vi "Trust Actual Server Identity.vi"(8 "error in (no error)":errorcluster, 10 "fingerprint":string, 11 "SSH Client in":refnum<class "OpenSSH Client.lvclass">) -> (0 "error out":errorcluster, 2 "permanent?":bool, 3 "SSH Client out":refnum<class "OpenSSH Client.lvclass">)   [LabVIEW 2020, in "NI_SSH.lvlib" / "OpenSSH Client.lvclass"]
uses:
  <vilib>/net/SSH/Client/OpenSSH/OpenSSH Client.lvclass
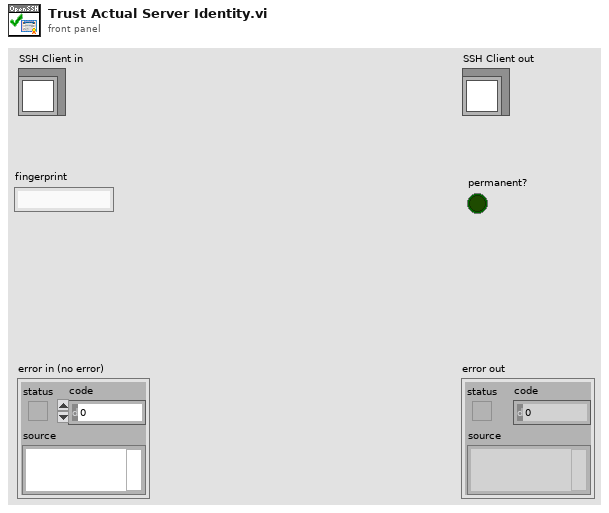
[diagram p1: front panel]
types:
  T1 = enum16{"open", "replace", "create", "open or create", "replace or create", "replace or create with confirmation"}
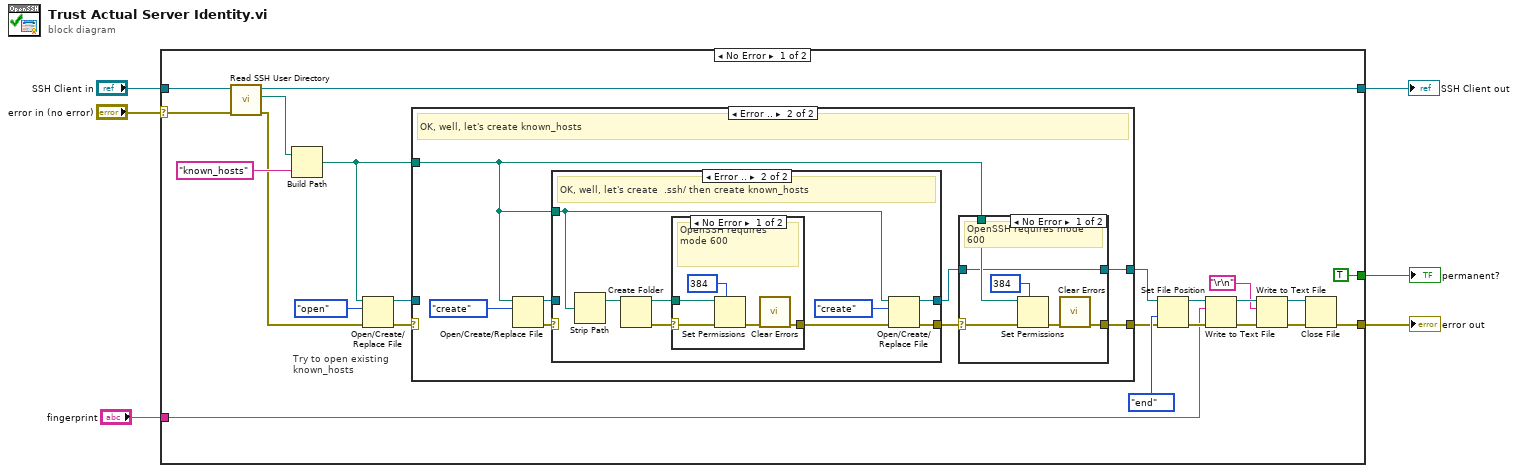
[diagram p0: block diagram]
diagram:
  n1 = case shown="No Error" "error in (no error)" {
    selector: "error in (no error)" -> [w28 w64]
    tunnel: "SSH Client in" -> [w29 w65]
    tunnel: "fingerprint" -> [w21 _]
    tunnel: [w15 w64] -> w3
    tunnel: [TRUE ("permanent?") _] -> w2
    tunnel: [w13 w65] -> w1
    frame No Error {
      # "Try to open existing known_hosts"
      n2 = call <vilib>:"Read SSH User Directory.vi"("error in (no error)"=w28, "OpenSSH Client in"=w29) -> ("error out"=w7:errorcluster, "Path"=w27:path, "OpenSSH Client out"=w13:refnum<class "OpenSSH Client.lvclass">)  [unwired: 7 in]
      n3 = Build Path(base path=w27, name or relative path="known_hosts") -> (appended path=w8:path)
      n4 = Open/Create/Replace File(file path (use dialog)=w8, error in=w7, operation (0:open)=T1."open") -> (refnum out=w11:refnum<file>, error out=w12:errorcluster)  [unwired: 3 in, 1 out]
      n5 = case shown="Error .." w12 {
        selector: w12 -> [w30 _]
        tunnel: w11 -> [w31 _]
        tunnel: [w31 w33] -> w9
        tunnel: [w30 w34] -> w10
        tunnel: w8 -> [_ w32]
        frame No Error {
        }
        frame Error {
          # "OK, well, let's create known_hosts"
          n6 = Open/Create/Replace File(file path (use dialog)=w32, operation (0:open)=T1."create") -> (refnum out=w37:refnum<file>, error out=w38:errorcluster)  [unwired: 4 in, 1 out]
          n7 = case shown="Error .." w38 {
            selector: w38 -> [w49 _]
            tunnel: [w49 w50] -> w35
            tunnel: w37 -> [w48 _]
            tunnel: [w48 w51] -> w36
            tunnel: w32 -> [_ w53]
            frame No Error {
            }
            frame Error {
              # "OK, well, let's create  .ssh/ then create known_hosts"
              n8 = Strip Path(path=w53) -> (stripped path=w57:path)  [unwired: 1 out]
              n9 = Create Folder(path (use dialog)=w57) -> (created path=w55:path, error out=w56:errorcluster)  [unwired: 2 in, 1 out]
              n10 = case shown="No Error" w56 {
                selector: w56 -> [w60 w63]
                tunnel: w55 -> [w61 _]
                tunnel: [w58 w63] -> w54
                frame No Error {
                  # "OpenSSH requires mode 600"
                  n11 = Set Permissions(7:i16 384 ("permissions"), 8:w60, 11:w61) -> (0:w59:errorcluster)  [unwired: 2 in, 1 out]
                  n12 = call <vilib>:"Clear Errors.vi"("error in (no error)"=w59) -> ("error out"=w58:errorcluster)  [unwired: 5 in, 1 out]
                }
                frame Error {
                  # "Well, phooey"
                }
              }
              n13 = Open/Create/Replace File(file path (use dialog)=w53, error in=w54, operation (0:open)=T1."create") -> (refnum out=w51:refnum<file>, error out=w50:errorcluster)  [unwired: 3 in, 1 out]
            }
          }
          n14 = case shown="No Error" w35 {
            selector: w35 -> [w45 w46]
            tunnel: [w41 w46] -> w34
            tunnel: w36 -> [w40 w47]
            tunnel: [w40 w47] -> w33
            tunnel: w32 -> [w44 _]
            frame No Error {
              # "OpenSSH requires mode 600"
              n15 = Set Permissions(7:i16 384 ("permissions"), 8:w45, 11:w44) -> (0:w42:errorcluster)  [unwired: 2 in, 1 out]
              n16 = call <vilib>:"Clear Errors.vi"("error in (no error)"=w42) -> ("error out"=w41:errorcluster)  [unwired: 5 in, 1 out]
            }
            frame Error {
            }
          }
        }
      }
      n17 = Set File Position(refnum=w9, from (0:start)=enum16{"start", "end", "current"}."end", error in=w10) -> (refnum out=w23:refnum<file>, error out=w22:errorcluster)  [unwired: 1 in]
      n18 = Write to Text File(file (use dialog)=w23, text=w21, error in=w22) -> (refnum out=w19:refnum<file>, error out=w20:errorcluster)  [unwired: 1 in, 1 out]
      n19 = Write to Text File(file (use dialog)=w19, text="\r\n", error in=w20) -> (refnum out=w16:refnum<file>, error out=w17:errorcluster)  [unwired: 1 in, 1 out]
      n20 = Close File(refnum=w16, error in=w17) -> (error out=w15:errorcluster)  [unwired: 1 out]
    }
    frame Error {
    }
  }
  "error out" <- w3
  "SSH Client out" <- w1
  "permanent?" <- w2
